vi "MKS946_Global.vi"() -> ()   [LabVIEW 2019]
panel:
  out "MKS946_P2":dbl
  out "MKS946_ST":u32(colorbox)
  out "MKS946_P1":dbl
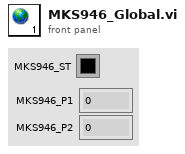
[diagram p1: front panel]
diagram:
